vi "Main.vi"() -> ()   [LabVIEW 2018]
uses:
  Consumer Message.ctl
panel:
  out "State to Execute":string
  out "High Priority?":bool
  out "Backlog":u8(slide) scale=0.0..100.0
  out "Processed Value":i32
  in  "High Priority Message":bool
  in  "Normal Priority Message":bool
  in  "Stop":bool
  # "Number of enqueued\nmessages waiting to\nbe processed"
  # "Current data being\nprocessed in consumer loop"
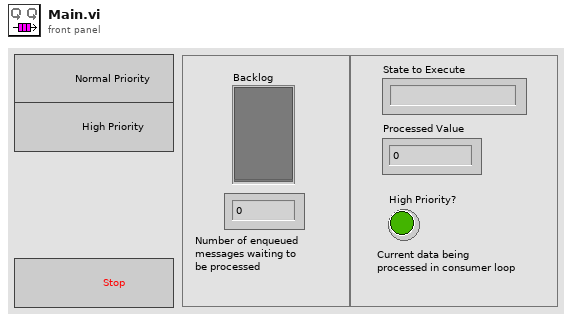
[diagram p1: front panel]
types:
  T1 = typedef "Consumer Message.ctl" = cluster{"Consumer State":string, "Boolean Data":bool, "Numeric Data":i32}
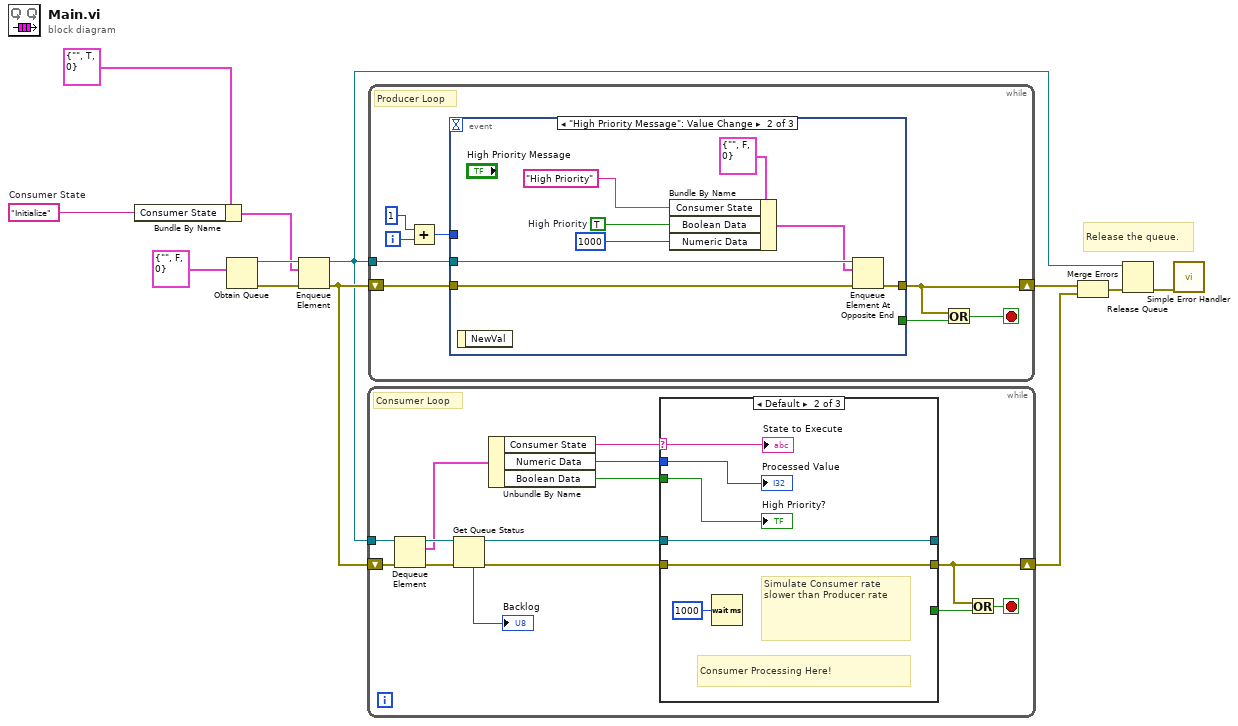
[diagram p0: block diagram]
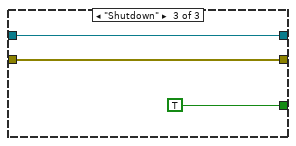
[diagram p3: hidden frame]
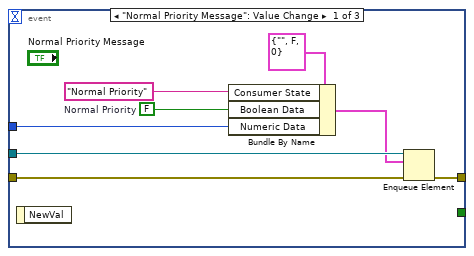
[diagram p4: hidden frame]
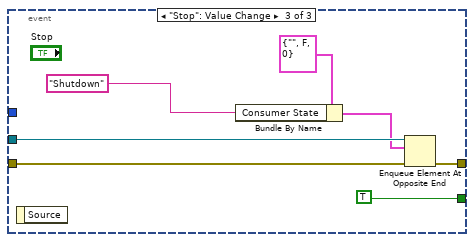
[diagram p5: hidden frame]
diagram:
  w1 = "Initialize"  # Consumer State
  # "Release the queue."
  n1 = Bundle By Name(cluster=T1 {"Consumer State"="", "Boolean Data"=TRUE, "Numeric Data"=0} ("Consumer Message"), "Consumer State"=w1) -> (w2:T1)
  n2 = Obtain Queue(element data type=T1 {"Consumer State"="", "Boolean Data"=FALSE, "Numeric Data"=0}) -> (queue out=w6:refnum<queue>, error out=w12:errorcluster)  [unwired: 4 in, 1 out]
  n3 = Enqueue Element(queue=w6, element=w2, error in (no error)=w12) -> (queue out=w5:refnum<queue>, error out=w7:errorcluster)  [unwired: 1 in, 1 out]
  n4 = while {
    tunnel: w5 -> [w24]
    shift-right: [w13] -> w11
    shift-left: w7 -> [w23]
    stop <- w14 stop-if-true
    # "Consumer Loop"
    n5 = Dequeue Element(queue=w24, error in (no error)=w23) -> (queue out=w25:refnum<queue>, element=w22:T1, error out=w26:errorcluster)  [unwired: 1 in, 1 out]
    n6 = Get Queue Status(queue=w25, error in (no error)=w26) -> (queue out=w16:refnum<queue>, error out=w20:errorcluster, # elements in queue=→"Backlog":i32)  [unwired: 1 in, 5 out]
    n7 = Unbundle By Name(w22) -> ("Consumer State"=w21:string, "Numeric Data"=w19:i32, "Boolean Data"=w17:bool)
    n8 = case shown="Default" w21 {
      selector: w21 -> [_ w31 _]
      tunnel: [_ _ TRUE] -> w15
      tunnel: w20 -> [w27 w29 w35]
      tunnel: [w27 w29 w35] -> w13
      tunnel: w19 -> [_ w34 _]
      tunnel: w17 -> [_ w33 _]
      tunnel: w16 -> [w28 w32 w36]
      tunnel: [w28 w32 w36] -> _
      frame "Initialize" {
      }
      frame Default {
        # "Simulate Consumer rate slower than Producer rate"
        # "Consumer Processing Here!"
        n9 = Wait (ms)(milliseconds to wait=u32 1000) -> ()  [unwired: 1 out]
        "Processed Value" <- w34
        "High Priority?" <- w33
        "State to Execute" <- w31
      }
      frame "Shutdown" {
      }
    }
    n10 = Or(x=w13, y=w15) -> (x .or. y?=w14:bool)
  }
  n11 = while {
    shift-right: [w41] -> w10
    shift-left: w7 -> [w44]
    tunnel: w5 -> [w45]
    i -> [w40]
    stop <- w42 stop-if-true
    # "Producer Loop"
    n12 = Add(x=1, y=w40) -> (x+y=w39:i32)
    n13 = event shown="[1] \"High Priority Message\": Value Change" {
      selector: _ -> [_ _ _]
      dyn-events: _ -> [_ _ _]
      timeout: _ -> [_ _ _]
      tunnel: w45 -> [w53 w60 w68]
      tunnel: w44 -> [w51 w59 w66]
      tunnel: [w52 w61 w65] -> w41
      tunnel: [_ _ TRUE] -> w43
      tunnel: w39 -> [w50 _ _]
      event "Normal Priority Message": Value Change {
        w47 = FALSE  # Normal Priority
        n14 = event-data() -> ()  [unwired: 1 in, 1 out]
        n15 = Bundle By Name(cluster=T1 {"Consumer State"="", "Boolean Data"=FALSE, "Numeric Data"=0}, "Consumer State"="Normal Priority" ("String Data"), "Boolean Data"=w47, "Numeric Data"=w50) -> (w49:T1)
        n16 = Enqueue Element(queue=w53, element=w49, error in (no error)=w51) -> (error out=w52:errorcluster)  [unwired: 1 in, 2 out]
      }
      event "High Priority Message": Value Change {
        w55 = TRUE  # High Priority
        n17 = event-data() -> ()  [unwired: 1 in, 1 out]
        n18 = Bundle By Name(cluster=T1 {"Consumer State"="", "Boolean Data"=FALSE, "Numeric Data"=0}, "Consumer State"="High Priority" ("String Data"), "Boolean Data"=w55, "Numeric Data"=1000) -> (w57:T1)
        n19 = Enqueue Element At Opposite End(queue=w60, element=w57, error in (no error)=w59) -> (error out=w61:errorcluster)  [unwired: 1 in, 2 out]
      }
      event "Stop": Value Change {
        n20 = event-data() -> ()  [unwired: 1 in, 1 out]
        n21 = Bundle By Name(cluster=T1 {"Consumer State"="", "Boolean Data"=FALSE, "Numeric Data"=0}, "Consumer State"="Shutdown") -> (w62:T1)
        n22 = Enqueue Element At Opposite End(queue=w68, element=w62, error in (no error)=w66) -> (error out=w65:errorcluster)  [unwired: 1 in, 2 out]
      }
    }
    n23 = Or(x=w41, y=w43) -> (x .or. y?=w42:bool)
  }
  n24 = Merge Errors(w10, w11) -> (w9:errorcluster)
  n25 = Release Queue(queue=w5, error in (no error)=w9) -> (error out=w4:errorcluster)  [unwired: 1 in, 2 out]
  n26 = call <vilib>:"Simple Error Handler.vi"("error in (no error)"=w4) -> ()  [unwired: 4 in, 5 out]
